vi "Initialise.vi"(8 "error in (no error)":errorcluster, 10 "Message in":refnum<class "InitialiseMessage.lvclass">, 11 "AOTF in":refnum<class "AOTF.lvclass">) -> (0 "error out":errorcluster, 3 "AOTF out":refnum<class "AOTF.lvclass">)   [LabVIEW 2012, in "AOTF.lvclass"]
doc: "This method is called when an initialise message is received. It mainly initialises the RabbitMQ connectivity. \n\nOverride this method when your component needs special initialisation (e.g. of software or hardware resources). In that case, don't forget to call the parent for proper implementation. If your component owns subcomponents, they count as resources, so you have to initialise them by calling their own initialise functions"
uses:
  AOTF.lvclass
  <vilib>/Distrio/Murmex/Murmex/Murmex.lvclass
  <vilib>/DAQmx/create/channels.llb/DAQmx Create Channel (DO-Digital Output).vi
  <vilib>/DAQmx/create/channels.llb/DAQmx Create Channel (AO-Voltage-Basic).vi
  <vilib>/Distrio/Murmex/InitialiseMessage/InitialiseMessage.lvclass
panel:
  # "This method is called when the INTIALISE\ntrigger is sent. \n\nOverride this method when your component needs to\nrespond to this trigger. \n\nCall parent for proper implementation"
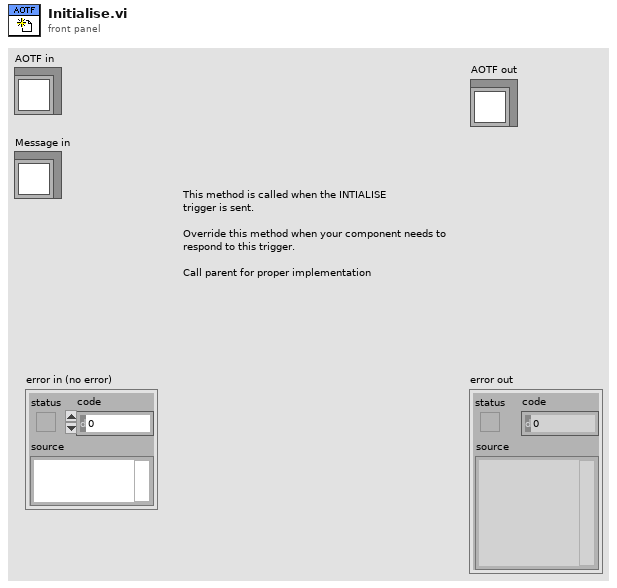
[diagram p1: front panel]
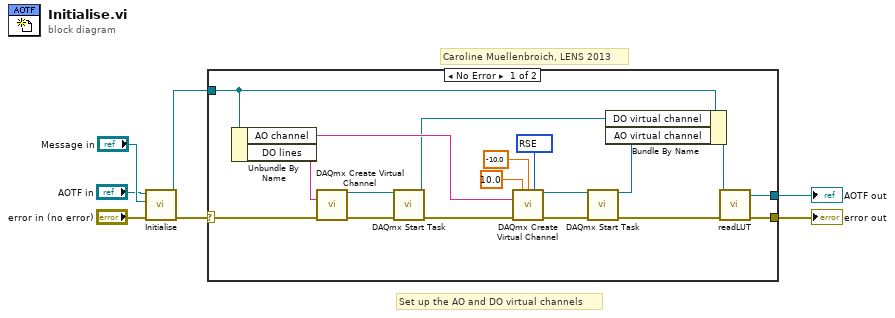
[diagram p0: block diagram]
diagram:
  # "Set up the AO and DO virtual channels"
  # "Caroline Muellenbroich, LENS 2013"
  n1 = call-parent "Initialise.vi"("error in (no error)"="error in (no error)", "Message in"="Message in", "Murmex in"="AOTF in") -> ("error out"=w4:errorcluster, "Murmex out"=w3:refnum<class "AOTF.lvclass">)  [unwired: 7 in]
  n2 = case shown="No Error" w4 {
    selector: w4 -> [w21 w27]
    tunnel: w3 -> [w22 w26]
    tunnel: [w25 w27] -> w2
    tunnel: [w23 w26] -> w1
    frame No Error {
      w18 = 10083 items=["Default"=-1, "RSE"=10083, "Differential"=10106, "Pseudodifferential"=12529] ("output terminal configuration")
      n3 = Unbundle By Name(w22) -> ("AO channel"=w19:tag, "DO lines"=w20:tag)
      n4 = call-poly <vilib>:"DAQmx Create Virtual Channel.vi"("lines"=w20, "error in"=w21) -> ("task out"=w13:refnum<k21>, "error out"=w15:errorcluster)  [unwired: 12 in]
      n5 = call <vilib>:"DAQmx Start Task.vi"("task/channels in"=w13, "error in"=w15) -> ("task out"=w12:refnum<k21>, "error out"=w14:errorcluster)  [unwired: 12 in]
      n6 = call-poly <vilib>:"DAQmx Create Virtual Channel.vi"("maximum value"=10.0, "minimum value"=-10.0, "output terminal configuration"=w18, "physical channels"=w19, "error in"=w14) -> ("task out"=w9:refnum<k21>, "error out"=w11:errorcluster)  [unwired: 9 in]
      n7 = call <vilib>:"DAQmx Start Task.vi"("task/channels in"=w9, "error in"=w11) -> ("task out"=w8:refnum<k21>, "error out"=w10:errorcluster)  [unwired: 12 in]
      n8 = Bundle By Name(cluster=w22, "DO virtual channel"=w12, "AO virtual channel"=w8) -> (w24:refnum<class "AOTF.lvclass">)
      n9 = call-dynamic "readLUT.vi"("error in (no error)"=w10, "AOTF in"=w24) -> ("error out"=w25:errorcluster, "AOTF out"=w23:refnum<class "AOTF.lvclass">)  [unwired: 8 in]
    }
    frame Error {
    }
  }
  "error out" <- w2
  "AOTF out" <- w1
